vi "From Variant.vi"(0 "Obj in":refnum<class "FSM.Node.lvclass">, 7 "Variant":variant, 9 "Prefix":string, 11 "error in (no error)":errorcluster) -> (4 "Obj out":refnum<class "FSM.Node.lvclass">, 15 "error out":errorcluster)   [LabVIEW 2020, in "FSM.Node.lvclass"]
uses:
  FSM.Node.lvclass
  FSM.Node.lvclass/FSM.Node.ctl
  epl-vi-lib/Koop/KObject Class/KObject.lvclass
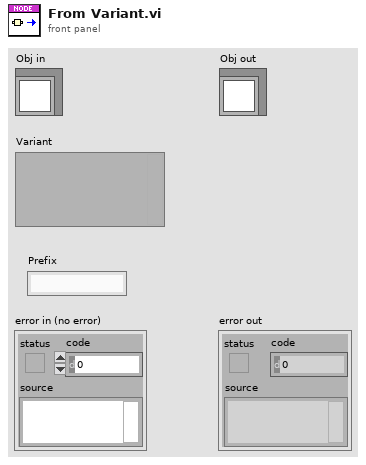
[diagram p1: front panel]
types:
  T1 = typedef "FSM.Node.lvclass/Serialized.ctl" = cluster{"Name":string, "BannerColor":u32, "Width":dbl, "Height":dbl, "FontSize":dbl, "Center":cluster{"X":dbl, "Y":dbl}, "Shape":T2, "Badges":T3[]}
  T2 = typedef "FSM.Node.lvclass/Shape.ctl" = enum16{"Default", "Start", "Action", "End"}
  T3 = typedef "FSM.Node.lvclass/Badge.ctl" = enum16{"Audio", "Visual"}
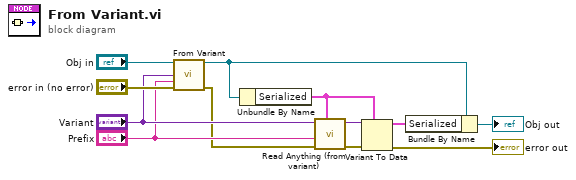
[diagram p0: block diagram]
diagram:
  n1 = call-parent "From Variant.vi"("KObject in"="Obj in", "Variant"="Variant", "Prefix"="Prefix", "error in (no error)"="error in (no error)") -> ("KObject out"=w3:refnum<class "FSM.Node.lvclass">, "error out"=w4:errorcluster)  [unwired: 10 in]
  n2 = Unbundle By Name(w3) -> ("Serialized"=w8:T1)
  n3 = call "Read Anything (from variant).vi"("Type of Anything"=w8, "Error In"=w4, "Prefix"="Prefix", "Variant Database"="Variant") -> ("Error Out"=w9:errorcluster, "Anything"=w10:variant)  [unwired: 5 in, 1 out]
  n4 = Variant To Data(error in=w9, type=w8, Variant=w10) -> (data=w7:T1, error out=→"error out":errorcluster)
  n5 = Bundle By Name(cluster=w3, "Serialized"=w7) -> (→"Obj out":refnum<class "FSM.Node.lvclass">)
